vi "Create ErrorMessage.vi"(8 "error in (no error)":errorcluster, 10 "Error Cluster":errorcluster, 11 "Message Name":string) -> (0 "error out":errorcluster, 3 "ErrorMessage out":refnum<class "ErrorMessage.lvclass">)   [LabVIEW 2009, in "LapDog.Messaging.v2.lvlib" / "ErrorMessage.lvclass"]
doc: "Creates an ErrorMessage object with the given name. If no name is given the message name is the same as the class name.\n\nThis method executes regardless of the error in state."
uses:
  ErrorMessage.lvclass
  MessageObject/Message.lvclass
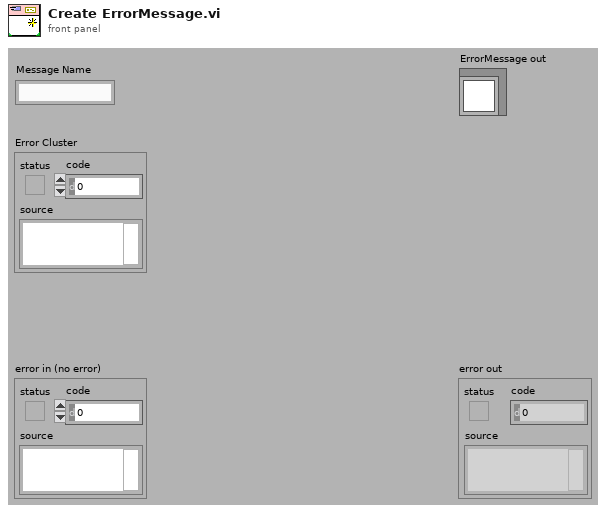
[diagram p1: front panel]
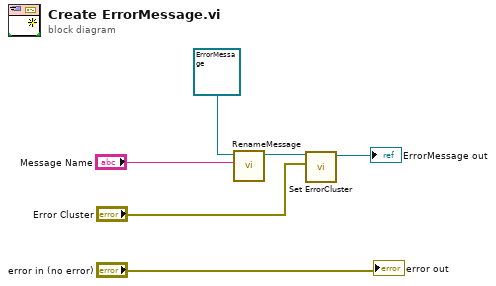
[diagram p0: block diagram]
diagram:
  n1 = call "RenameMessage.vi"("Message Name"="Message Name", "Message in"=refnum<class "ErrorMessage.lvclass"> refnum ("ErrorMessage in")) -> ("Message out"=w3:refnum<class "ErrorMessage.lvclass">)  [unwired: 8 in, 1 out]
  n2 = call-dynamic "Set ErrorCluster.vi"("ErrorCluster"="Error Cluster", "ErrorMessage"=w3) -> ("ErrorMessage out"=→"ErrorMessage out":refnum<class "ErrorMessage.lvclass">)  [unwired: 8 in, 1 out]
  "error out" <- "error in (no error)"
